vi "LSL Array buildup.vi"() -> ()   [LabVIEW 2016]
panel:
  out "output array":dbl[][](array[numeric])
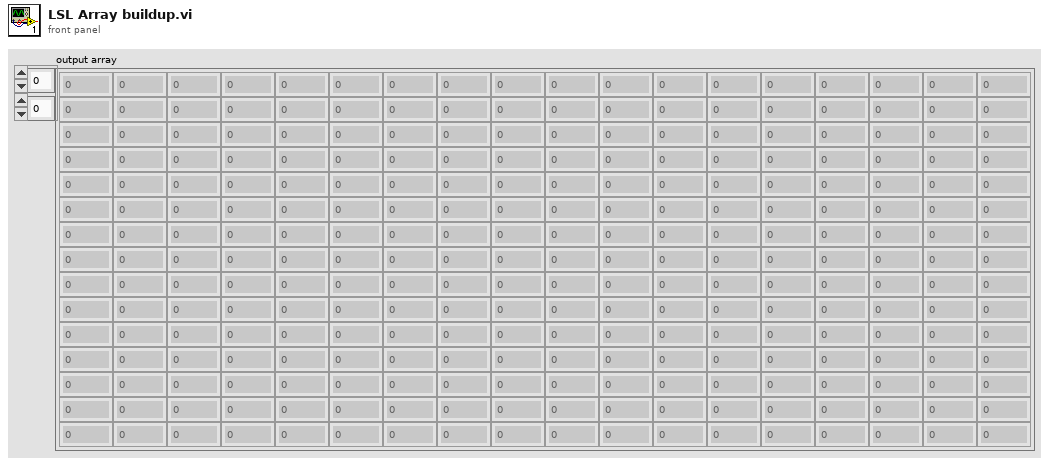
[diagram p1: front panel]
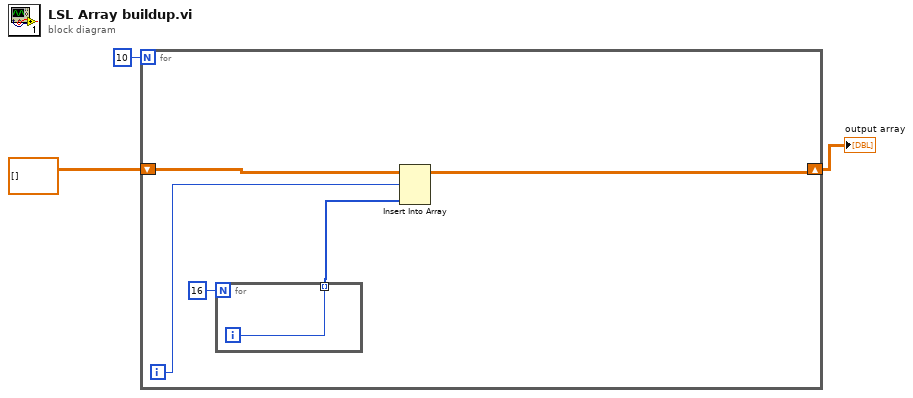
[diagram p0: block diagram]
diagram:
  n1 = for {
    N: 10 -> [_]
    shift-right: [w4] -> w1
    shift-left: dbl[][] [] -> [w8]
    i -> [w5]
    n2 = for {
      N: 16 -> [_]
      tunnel: [w9] -> w6 mode=indexing
      i -> [w9]
    }
    n3 = Insert Into Array(array=w8, index (row)=w5, new element=w6) -> (w4:dbl[][])  [unwired: 1 in]
  }
  "output array" <- w1
